vi "preview_popup.vi"(6 "var mode":enum16{"permutations", "aligned"}(ring), 8 "v1_values":dbl[](array[numeric])=[0.0] format="%#_6p", 9 "v1_config":T1={"hardware"=enum."none", "options"="", "repeats"=1, "loops"=4, "VISA"="", "override_VISA"=FALSE} {"loops" min=1; "repeats" min=1}, 10 "v0_values":dbl[](array[numeric]) format="%#_6p", 11 "v0_config":T1={"hardware"=enum."wf_multi_freq", "options"="", "repeats"=6, "loops"=1, "VISA"="", "override_VISA"=FALSE} {"loops" min=1; "repeats" min=1}) -> (1 "rows":i32, 2 "scan_values":dbl[][](array[numeric]) format="%#_6p")   [LabVIEW 2017, in "tools.lvlib"]
uses:
  tools.lvlib
  core/var_config.ctl
  ctrl/var_list.ctl
panel:
  out "min v1":dbl
  out "max v1":dbl
  out "min v0":dbl
  out "max v0":dbl
  out "v1":dbl[](graph)
  out "v0":dbl[](graph)
  out "var mode 2":enum16{"permutations", "aligned"}(ring) caption="var mode"
  in  "OK":bool
  # "scan parameters"
  # "v0"
  # "v1"
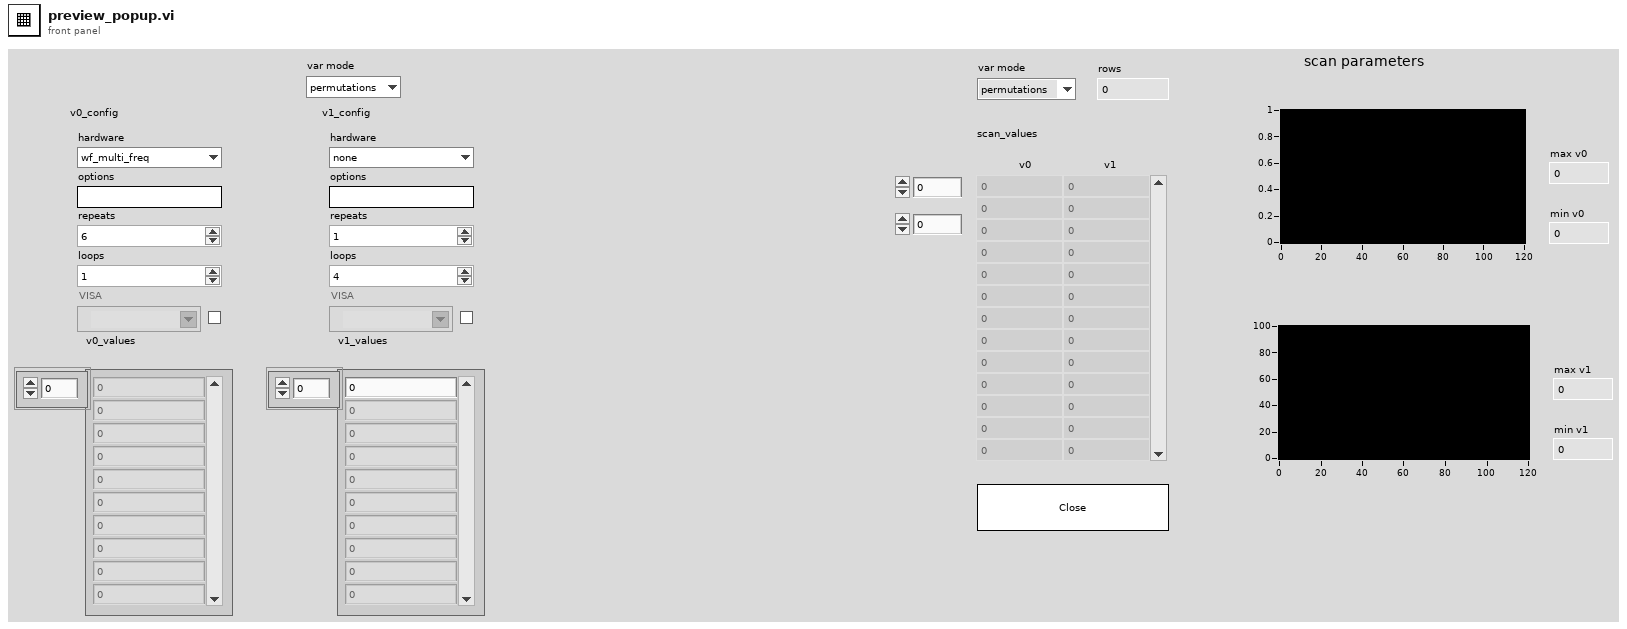
[diagram p1: front panel]
types:
  T1 = typedef "tools.lvlib/var_config.ctl" = cluster{"hardware":T2, "options":string, "repeats":i32, "loops":i32, "VISA":refnum<visa-resource-name>, "override_VISA":bool}
  T2 = typedef "var_list.ctl" = enum16{"none", "AO voltage (V)", "delay (s)", "generic", "microwaves (GHz)", "radiant (nm)", "radiant thg (nm)", "sirah (nm)", "sirah_shg (nm)", "tenma voltage (V)", "wait (s)", "wf_freq (Hz)", "wf_amp (V)", "wf_offset (V)", "wf_low_level (V)", "wf_high_level (V)", "wf_period (s)", "wf_pulse_width (s)", "wf_sample_rate (Sa/s)", "wf_multi_amp", "wf_multi_freq", "wf_arb_4chan", "WS7 setpoint (nm)"}
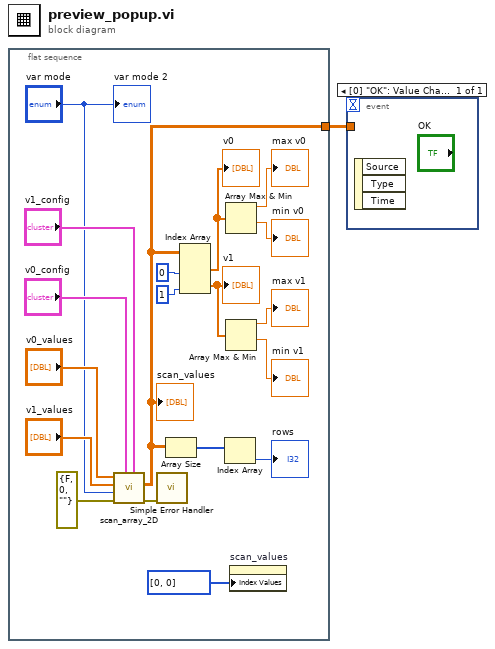
[diagram p0: block diagram]
diagram:
  n1 = flat-sequence {
    tunnel: [w11] -> w1
    frame #0 {
      n2 = call "scan_array_2D.vi"("v1_config"="v1_config", "v0_config"="v0_config", "error in"=errorcluster {"status"=FALSE, "code"=0, "source"=""}, "var mode"="var mode", "v1_values"="v1_values", "v0_values"="v0_values") -> ("error in (no error)"=w12:errorcluster, "scan_values"=w11:dbl[][])  [unwired: 4 in]
      "scan_values" <- w11
      n3 = call <vilib>:"Simple Error Handler.vi"("error in (no error)"=w12) -> ()  [unwired: 4 in, 5 out]
      n4 = Array Size(array=w11) -> (size(s)=w20:i32[])
      n5 = Index Array(array=w11, index (col) #1=0 ("disabled index (col)"), index (col) #2=1 ("index (col)")) -> (element #1=w8:dbl[], element #2=w5:dbl[])  [unwired: 2 in]
      "v0" <- w8
      "v1" <- w5
      n6 = Index Array(array=w20) -> (element=→"rows":i32)  [unwired: 1 in]
      n7 = Array Max & Min(array=w8) -> (max value=→"max v0":dbl, min value=→"min v0":dbl)  [unwired: 2 out]
      n8 = Array Max & Min(array=w5) -> (max value=→"max v1":dbl, min value=→"min v1":dbl)  [unwired: 2 out]
      n9 = property on="scan_values" class="Arr (strict)"("Index Values"=u32[] [0, 0]) -> ()  [unwired: 2 in, 2 out]
      "var mode 2" <- "var mode"
    }
  }
  n10 = event shown="[0] \"OK\": Value Change;  Panel Close" {
    selector: _ -> [_]
    dyn-events: _ -> [_]
    timeout: _ -> [_]
    tunnel: w1 -> [_]
    event "OK": Value Change; Panel Close {
      n11 = event-data() -> ()  [unwired: 1 in, 3 out]
    }
  }
